vi "rsmxo_LV2015_Fetch_Waveform_only_Example.vi"() -> ()   [LabVIEW 2015]
uses:
  <instrlib>/Rohde&Schwarz MXO Oscilloscopes/Rohde&Schwarz MXO Oscilloscopes.lvlib
panel:
  out "Waveform Graph":T1(graph)={"X Start"=-0.05, "X Start"=1.0000000000000002e-08, "Waveform Data"=array[100000 elements]}
  in  "Channel":i32(ring)=1 caption="Channel (1)" items=["1"=1, "2"=2, "3"=3, "4"=4, "External"=5]
  in  "VISA resource name":refnum<visa-resource-name>="TCPIP::10.205.0.159::hislip0"
  in  "Reset":bool
  in  "ID Query":bool=TRUE
  # "Rohde & Schwarz RTM2000 Oscilloscope Read Waveform Example"
  # "Rohde & Schwarz MXO Oscilloscopes Series\nFetch Waveform only Example"
  # "Before running, change the VISA resource name to fit your device:\n- For LAN interface use TCPIP::<IP_Address>::INSTR e.g. TCPIP::10.64.0.178::INSTR\n- For USB interface use USB0::0x0AAD::<PID>::<SN>::INSTR e.g. USB0::0x0AAD::0x01D6::101457::INSTR\n- For GPIB interface use the GPIB::<Address>::INSTR e.g. GPIB::28::INSTR"
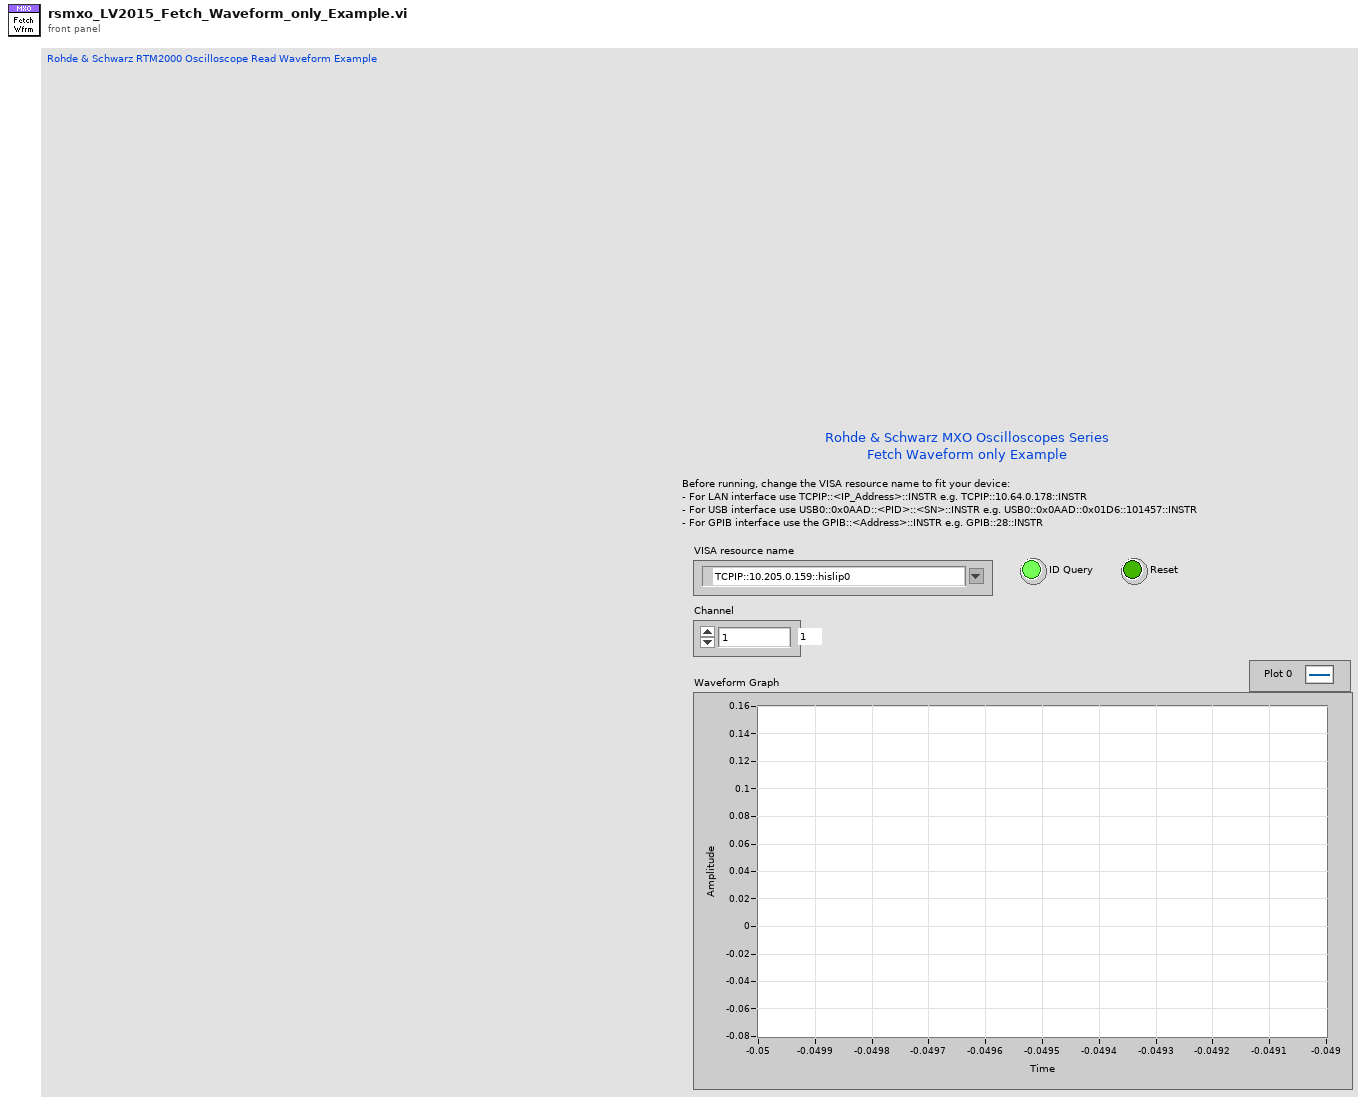
[diagram p1: front panel]
types:
  T1 = cluster{"X Start":dbl, "X Start":dbl, "Waveform Data":dbl[]}
  T2 = cluster{"X Start":dbl, dbl, "Waveform Data":dbl[]}
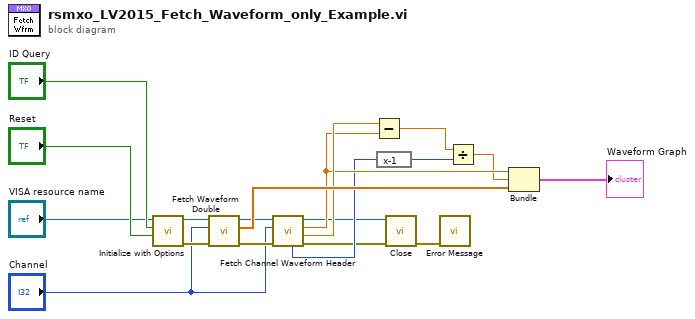
[diagram p0: block diagram]
diagram:
  n1 = call <instrlib>:"Initialize with Options.vi"("Reset (T: Reset)"="Reset", "ID Query (T: Check)"="ID Query", "VISA resource name"="VISA resource name") -> ("error out"=w8:errorcluster, "VISA resource name out"=w7:refnum<visa-resource-name>)  [unwired: 7 in]
  n2 = call <instrlib>:"Fetch Waveform Double.vi"("error in (no error)"=w8, "Source (Channel 1)"="Channel", "VISA resource name"=w7) -> ("error out"=w6:errorcluster, "Waveform Data"=w16:dbl[], "VISA resource name out"=w5:refnum<visa-resource-name>)  [unwired: 6 in]
  n3 = call <instrlib>:"Fetch Channel Waveform Header.vi"("error in (no error)"=w6, "Channel (1)"="Channel", "VISA resource name"=w5) -> ("error out"=w4:errorcluster, "X Stop"=w14:dbl, "X Start"=w13:dbl, "VISA resource name out"=w3:refnum<visa-resource-name>, "Record Length"=w11:i32)  [unwired: 3 in, 1 out]
  n4 = Subtract(x=w14, y=w13) -> (x-y=w12:dbl)
  n5 = expression code="x-1"(w11) -> (w10:i32)
  n6 = call <instrlib>:"Close.vi"("error in (no error)"=w4, "VISA resource name"=w3) -> ("error out"=w2:errorcluster)  [unwired: 9 in]
  n7 = call <instrlib>:"Error Message.vi"("error in (no error)"=w2) -> ()  [unwired: 10 in, 5 out]
  n8 = Divide(x=w12, y=w10) -> (x/y=w9:dbl)
  n9 = Bundle("X Start"=w13, w9, "Waveform Data"=w16) -> (→"Waveform Graph":T2)  [unwired: 1 in]
